vi "Stop Core.vi"(10 "final error code":i32, 11 "CS++MCS in":refnum<class "CS++MCS.lvclass">) -> (3 "CS++MCS out":refnum<class "CS++MCS.lvclass">)   [LabVIEW 2016, in "CS++MCS.lvlib" / "CS++MCS.lvclass"]
doc: "(<B>Filename</B>: Actor Framework.lvlib:Actor.lvclass:Stop Core.vi)\n\nDefines what the actor does before it stops. Use the <B>final error code</B> input to determine whether the actor shut down in response to an error.\n\nBy default, this method does nothing. A descendant class may override it to define behavior, such as shutting down any processes the actor initiated in its override of the Actor Core method."
uses:
  CS++MCS.lvclass
  CS++MCS.lvclass/CS++MCS.ctl
  CSPP_Core/Actors/CS++DeviceActor/CS++DeviceActor.lvclass
  CSPP_Core/Classes/CS++ProcessVariables/PVConnection/PVConnection.lvclass
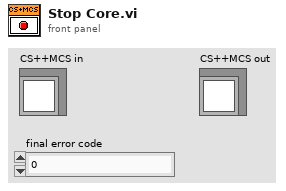
[diagram p1: front panel]
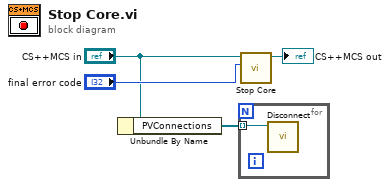
[diagram p0: block diagram]
diagram:
  n1 = Unbundle By Name("CS++MCS in") -> ("PVConnections"=w1:refnum<class "PVConnection.lvclass">[])
  n2 = for {
    tunnel: w1 -> [w5] mode=indexing
    n3 = call "Disconnect.vi"("PVConnection in"=w5) -> ()  [unwired: 9 in, 2 out]
  }
  n4 = call-parent "Stop Core.vi"("final error code"="final error code", "CS++DeviceActor in"="CS++MCS in") -> ("CS++DeviceActor out"=→"CS++MCS out":refnum<class "CS++MCS.lvclass">)  [unwired: 9 in]
